vi "Initial Data Save.vi"(8 "error in (no error)":errorcluster, 9 "index":i32=30, 10 "OK and NG":bool, 11 "String In":string="$AGENT.81,C8.C8,S*03") -> (0 "error out":errorcluster)   [LabVIEW 2019]
uses:
  Ctrl/MeasureDisplayTab.ctl
  Ctrl/Table Save.ctl
  LLB/Commonly VI/Main Glb.vi
  Global/Process Global.vi
  LLB/Commonly VI.lvlib
panel:
  out "機種廠商代號":string
  out "硬體版本":string
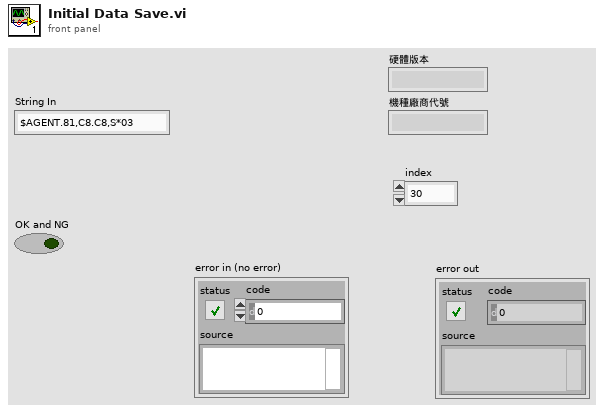
[diagram p1: front panel]
types:
  T1 = typedef "Table Save.ctl" = enum16{"initial", "Add", "Write", "Replace", "Delete", "REad", "RedTable", "Load"}
  T2 = typedef "MeasureDisplayTab.ctl" = enum16{"Tray Barcode", "PCBA BARCODE", "硬體(Tool初始化)", "company(Tool初始化)", "耗電流 uA(電流表)", "電池負載電壓", "晶片ID(Tool FORMAT)", "雷雕ID(TOOl scan、藍芽接收器)", "Format(Tool FORMAT)", "Programe(Tool Programe)", "MAC(藍芽接收器)", "ID(藍芽接收器)", "KPA(藍芽接收器)", "溫度(藍芽接收器)", "SENSOR電池電壓(藍芽接收器)", "RSSI(藍芽接收器)", "SensorType_315(FSK scan)", "FSKsnVol_315(FSK scan)", "FSKscanl_315(FSK scan)", "P_315(FSK scan)", "T_315(FSK scan)", "SensorType_433(ASK scan)", "ASKsnVol_433(ASK scan)", "ASKscan_433(ASK scan)", "P_433(ASK scan)", "T_433(ASK scan)", "測高Data"}
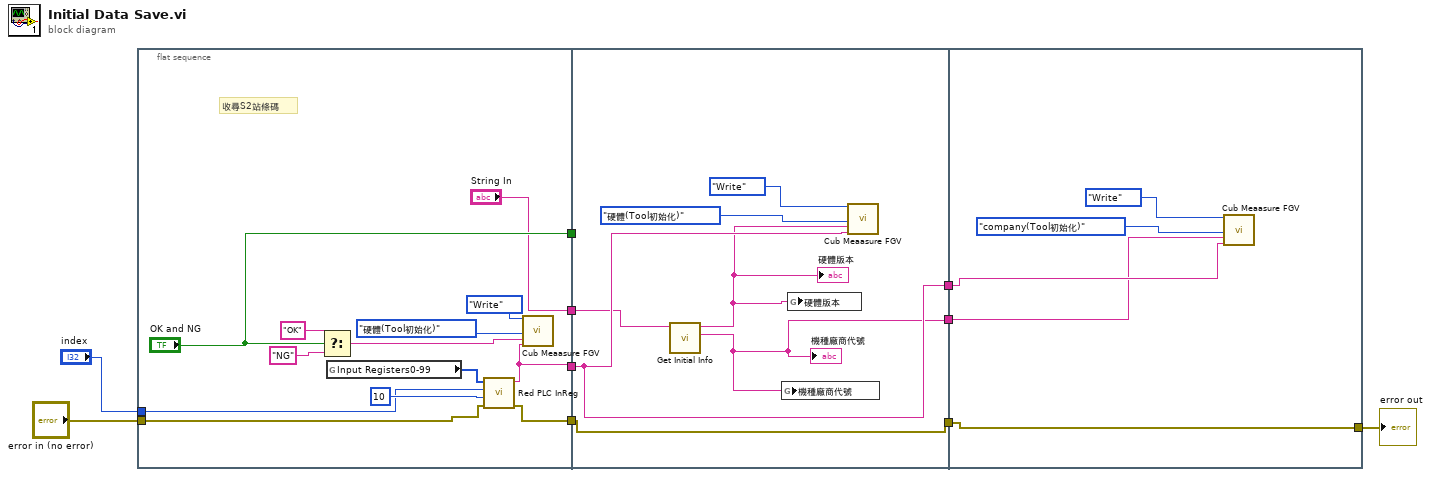
[diagram p0: block diagram]
diagram:
  n1 = flat-sequence {
    tunnel: [w16] -> w10
    tunnel: ["OK and NG"] -> w7
    tunnel: "error in (no error)" -> [w12]
    tunnel: [w11] -> w4
    tunnel: ["String In"] -> w2
    tunnel: "index" -> [w13]
    tunnel: w10 -> [w29]
    tunnel: [w29] -> w9
    tunnel: [w25] -> w8
    tunnel: w7 -> [_]
    tunnel: [w30] -> w5
    tunnel: w4 -> [w30]
    tunnel: w2 -> [w28]
    tunnel: w9 -> [w33]
    tunnel: w8 -> [w32]
    tunnel: w5 -> [w31]
    tunnel: [w31] -> w3
    frame #0 {
      # "收尋S2站條碼"
      n2 = Select(t="OK" ("DataIn"), s="OK and NG", f="NG" ("DataIn")) -> (s? t:f=w23:string)
      n3 = global read "Main Glb.vi" "Input Registers0-99"() -> (w17:u16[])
      n4 = call "Red PLC InReg.vi"("error in (no error)"=w12, "length"=10, "index"=w13, "Input Registers Arr"=w17) -> ("error out"=w11:errorcluster, "Rad In Reg"=w16:string)  [unwired: 6 in]
      n5 = call "Cub Meaasure FGV.vi"("Action"=Table_Save."Write" ("Enum"), "Save Index"=MeasureDisplayTab."硬體(Tool初始化)", "DataIn"=w23, "SN"=w16) -> ()  [unwired: 8 in, 8 out]
    }
    frame #1 {
      n6 = call "Get Initial Info.vi"("String"=w28) -> ("機種廠商代號"=w25:string, "硬體版本"=w24:string)  [unwired: 9 in]
      "硬體版本" <- w24
      "機種廠商代號" <- w25
      n7 = global write "Process Global.vi" "機種廠商代號"(w25) -> ()
      n8 = global write "Process Global.vi" "硬體版本"(w24) -> ()
      n9 = call "Cub Meaasure FGV.vi"("Action"=Table_Save."Write" ("Enum"), "Save Index"=MeasureDisplayTab."硬體(Tool初始化)", "DataIn"=w24, "SN"=w29) -> ()  [unwired: 8 in, 8 out]
    }
    frame #2 {
      n10 = call "Cub Meaasure FGV.vi"("Action"=Table_Save."Write" ("Enum"), "Save Index"=MeasureDisplayTab."company(Tool初始化)", "DataIn"=w32, "SN"=w33) -> ()  [unwired: 8 in, 8 out]
    }
  }
  "error out" <- w3
